vi "Write Generated files.vi"(9 "ProjectItem in":refnum<class "ProjectItem.lvclass">, 10 "Generated files":path[](array[path]), 11 "BuildManager in":refnum<class "BuildManager.lvclass">) -> (3 "BuildManager out":refnum<class "BuildManager.lvclass">)   [LabVIEW 2019, in "SolutionBuilder.lvlib" / "BuildManager.lvclass"]
uses:
  BuildManager.lvclass
  ProjectItem/ProjectItem.lvclass
  BuildManager.lvclass/BuildManager.ctl
  <vilib>/Utility/miscctls.llb/LVMapReplaceAction.ctl
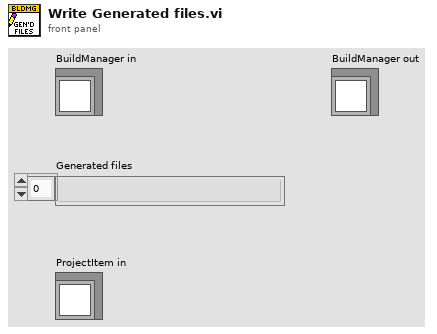
[diagram p1: front panel]
types:
  T1 = typedef "LVMapReplaceAction.ctl" = enum32{"Modify Entry only if found", "Add or Modify Entry", "Delete Entry"}
  T2 = typedef "SolutionBuilder.lvlib/BuildManager.lvclass/GeneratedFile.ctl" = map{cluster{"Project path":string, "Build spec name":string}, set{string}}
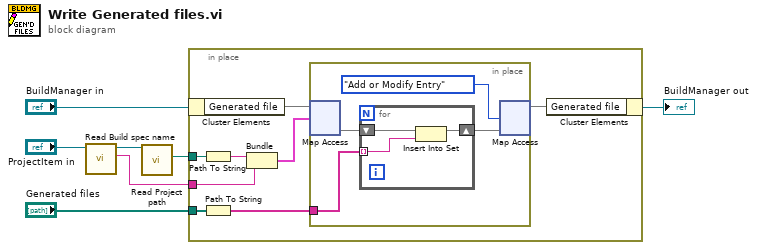
[diagram p0: block diagram]
diagram:
  n1 = call "Read Build spec name.vi"("ProjectItem in"="ProjectItem in") -> ("Build spec name"=w4:string, "ProjectItem out"=w5:refnum<class "ProjectItem.lvclass">)  [unwired: 9 in]
  n2 = call "Read Project path.vi"("ProjectItem in"=w5) -> ("Project path"=w3:path)  [unwired: 9 in, 1 out]
  n3 = in-place {
    in-place-border: "Generated files" -> [w8]
    in-place-border: w4 -> [w15]
    in-place-border: w3 -> [w14]
    n4 = in-place-cluster #1("BuildManager in") -> ("Generated file"=w13:T2)
    n5 = Path To String(path=w14) -> (string=w10:string)
    n6 = Path To String(path=w8) -> (string=w9:string[])
    n7 = Bundle(w10, "Build spec name"=w15) -> (w11:cluster{string, "Build spec name":string})  [unwired: 1 in]
    n8 = in-place {
      in-place-border: w9 -> [w17]
      n9 = in-place-map #2(w13, w11) -> (w19:set{string})  [unwired: 1 in, 1 out]
      n10 = for {
        shift-right: [w20] -> w18
        shift-left: w19 -> [w22]
        tunnel: w17 -> [w21] mode=indexing
        n11 = Insert Into Set(10:w21, 11:w22) -> (3:w20:set{string})  [unwired: 1 out]
      }
      n12 = in-place-map #2(w18, LVMapReplaceAction."Add or Modify Entry" ("action")) -> (w12:T2)  [unwired: 2 out]
    }
    n13 = in-place-cluster #1("Generated file"=w12) -> (→"BuildManager out":refnum<class "BuildManager.lvclass">)
  }
